vi "close data FIFOs.vi"(11 "Data FIFOs":T1) -> ()   [LabVIEW 2015, in "E2E Runtime (RT FIFO).lvclass"]
uses:
  E2E Runtime (RT FIFO).lvclass
  Data FIFOs.ctl
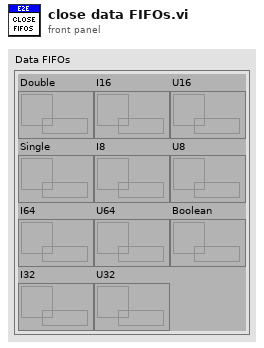
[diagram p1: front panel]
types:
  T1 = typedef "E2E Runtime (RT FIFO).lvclass/Data FIFOs.ctl" = cluster{"Double":refnum<k33>, "Single":refnum<k33>, "I64":refnum<k33>, "I32":refnum<k33>, "I16":refnum<k33>, "I8":refnum<k33>, "U64":refnum<k33>, "U32":refnum<k33>, "U16":refnum<k33>, "U8":refnum<k33>, "Boolean":refnum<k33>}
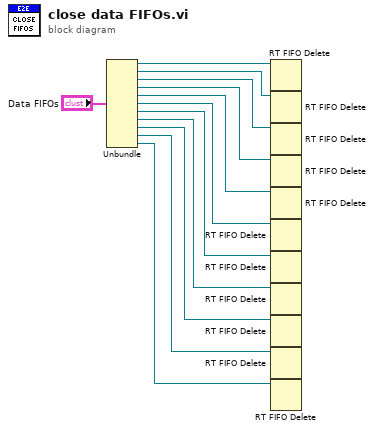
[diagram p0: block diagram]
diagram:
  n1 = Unbundle("Data FIFOs") -> ("Double"=w11:refnum<k33>, "Single"=w10:refnum<k33>, "I64"=w9:refnum<k33>, "I32"=w8:refnum<k33>, "I16"=w7:refnum<k33>, "I8"=w6:refnum<k33>, "U64"=w5:refnum<k33>, "U32"=w4:refnum<k33>, "U16"=w3:refnum<k33>, "U8"=w2:refnum<k33>, "Boolean"=w1:refnum<k33>)
  n2 = RT FIFO Delete(0:w11) -> ()  [unwired: 2 in, 1 out]
  n3 = RT FIFO Delete(0:w10) -> ()  [unwired: 2 in, 1 out]
  n4 = RT FIFO Delete(0:w9) -> ()  [unwired: 2 in, 1 out]
  n5 = RT FIFO Delete(0:w8) -> ()  [unwired: 2 in, 1 out]
  n6 = RT FIFO Delete(0:w7) -> ()  [unwired: 2 in, 1 out]
  n7 = RT FIFO Delete(0:w6) -> ()  [unwired: 2 in, 1 out]
  n8 = RT FIFO Delete(0:w5) -> ()  [unwired: 2 in, 1 out]
  n9 = RT FIFO Delete(0:w4) -> ()  [unwired: 2 in, 1 out]
  n10 = RT FIFO Delete(0:w3) -> ()  [unwired: 2 in, 1 out]
  n11 = RT FIFO Delete(0:w2) -> ()  [unwired: 2 in, 1 out]
  n12 = RT FIFO Delete(0:w1) -> ()  [unwired: 2 in, 1 out]
